vi "overlap_calculator.vi"(0 "T1":dbl, 2 "T2":dbl, 3 "D":dbl) -> (6 "overlap":dbl)   [LabVIEW 2015]
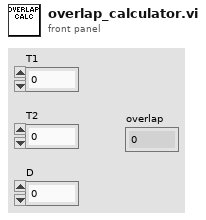
[diagram p1: front panel]
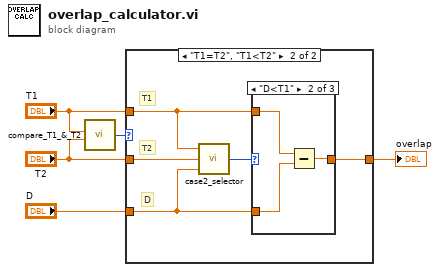
[diagram p0: block diagram]
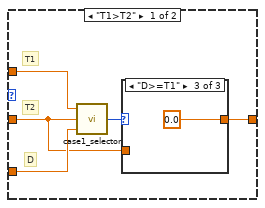
[diagram p2: hidden frame]
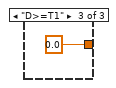
[diagram p6: hidden frame]
diagram:
  n1 = call "compare_T1_&_T2.vi"("T1"="T1", "T2"="T2") -> ("Result"=w1:enum16{"T1>T2", "T1=T2", "T1<T2"})  [unwired: 6 in]
  n2 = case shown="\"T1=T2\", \"T1<T2\"" w1 {
    tunnel: "T1" -> [w9 w16]
    tunnel: "T2" -> [w7 w18]
    tunnel: "D" -> [w10 w14]
    tunnel: [w6 w15] -> w5
    frame "T1>T2" {
      # "D"
      # "T2"
      # "T1"
      n3 = call "case1_selector.vi"("T1"=w9, "T2"=w7, "Delay"=w10) -> ("Case 1 selector"=w8:enum16{"D<=T1-T2", "T1-T2<D<T1", "D>=T1"})  [unwired: 4 in]
      n4 = case shown="\"D>=T1\"" w8 {
        tunnel: w7 -> [w11 w12 _]
        tunnel: [w11 w12 0.0] -> w6
        frame "D<=T1-T2" {
        }
        frame "T1-T2<D<T1" {
        }
        frame "D>=T1" {
        }
      }
    }
    frame "T1=T2", "T1<T2" {
      # "D"
      # "T2"
      # "T1"
      n5 = call "case2_selector.vi"("T1"=w16, "T2"=w18, "Delay"=w14) -> ("Case 2 selector"=w17:enum16{"D=0", "D<T1", "D>=T1"})  [unwired: 4 in]
      n6 = case shown="\"D<T1\"" w17 {
        tunnel: w16 -> [w19 w21 _]
        tunnel: [w19 w22 0.0] -> w15
        tunnel: w14 -> [_ w20 _]
        frame "D=0" {
        }
        frame "D<T1" {
          n7 = Subtract(x=w21, y=w20) -> (x-y=w22:dbl)
        }
        frame "D>=T1" {
        }
      }
    }
  }
  "overlap" <- w5
